vi "Initialization VI.vi"(8 "error in (no error)":errorcluster, 10 "Custom XML":string, 11 "Device Item Ref in":T1 format="%.0x") -> (0 "error out":errorcluster, 3 "Device Item Ref out":T1 format="%.0x")   [LabVIEW 2027, in "System Monitor System Explorer.lvlib"]
uses:
  System Monitor System Explorer.lvlib
  <vilib>/NI VeriStand/Custom Device API/Custom Device Item Ref.ctl
  Shared/System Monitor Settings.ctl
  Shared/System Monitor Shared.lvlib
  <vilib>/NI VeriStand/Custom Device API/Custom Device API.lvlib
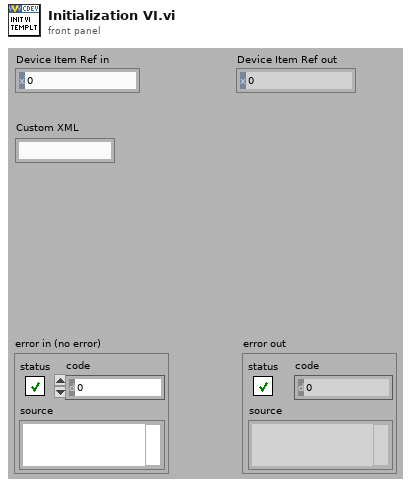
[diagram p1: front panel]
types:
  T1 = typedef "Custom Device API.lvlib/Custom Device Item Ref.ctl" = u64
  T2 = typedef "System Monitor Shared.lvlib/System Monitor Settings.ctl" = cluster{"Number of CPU Cores":u64, "Update Rate (Hz)":dbl}
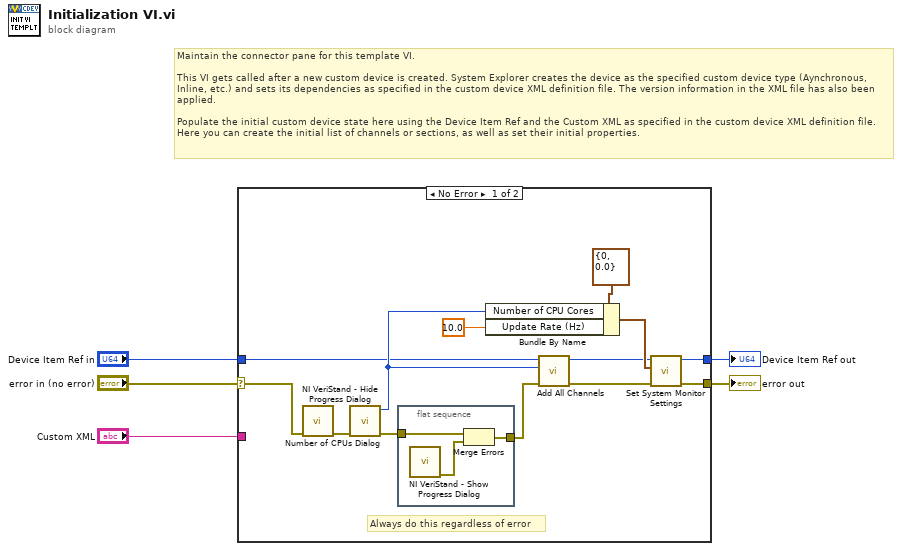
[diagram p0: block diagram]
diagram:
  # "Maintain the connector pane for this template VI.\n\nThis VI gets called after a new custom device is created. System Explorer creates the device as the specified custom device type (Aynchronous, Inline, etc.) and sets its dependencies as specified in the custom device XML definition file. The version information in the XML file has also been applied.\n\nPopulate the initial custom device state here using the Device Item Ref and the Custom XML as specified in the custom device XML definition file. Here you can create the initial list of channels or sections, as well as set their initial properties."
  n1 = case shown="No Error" "error in (no error)" {
    selector: "error in (no error)" -> [w9 w23]
    tunnel: [w13 w23] -> w5
    tunnel: [w14 w22] -> w3
    tunnel: "Device Item Ref in" -> [w10 w22]
    tunnel: "Custom XML" -> [_ _]
    frame No Error {
      # "Always do this regardless of error"
      n2 = call <vilib>:"NI VeriStand - Hide Progress Dialog.vi"("error in (no error)"=w9) -> ("error out"=w8:errorcluster)  [unwired: 10 in]
      n3 = call "Number of CPUs Dialog.vi"("error in (no error)"=w8) -> ("error out"=w7:errorcluster, "CPU_Cores"=w11:u64)  [unwired: 9 in]
      n4 = flat-sequence {
        tunnel: w7 -> [w21]
        tunnel: [w19] -> w6
        frame #0 {
          n5 = call <vilib>:"NI VeriStand - Show Progress Dialog.vi"() -> ("error out"=w20:errorcluster)  [unwired: 11 in]
          n6 = Merge Errors(w21, w20) -> (w19:errorcluster)
        }
      }
      n7 = Bundle By Name(cluster=T2 {"Number of CPU Cores"=0, "Update Rate (Hz)"=0.0} ("System Monitor Settings"), "Number of CPU Cores"=w11, "Update Rate (Hz)"=10.0) -> (w16:T2)
      n8 = call "Add All Channels.vi"("error in (no error)"=w6, "Number of CPU Cores in"=w11, "Item Ref in"=w10) -> ("error out"=w12:errorcluster, "Item Ref out"=w15:T1)  [unwired: 7 in]
      n9 = call "Set System Monitor Settings.vi"("error in (no error)"=w12, "System Monitor Settings"=w16, "Item Ref in"=w15) -> ("error out"=w13:errorcluster, "Item Ref out"=w14:T1)  [unwired: 7 in]
    }
    frame Error {
    }
  }
  "error out" <- w5
  "Device Item Ref out" <- w3
